vi "RDV-linkPlotSize.vi"(8 "error in (no error)":errorcluster, 11 "RDV-Reflection_Data_viewer in":refnum<class "RDV-Reflection_Data_viewer.lvclass">) -> (0 "error out":errorcluster, 3 "RDV-Reflection_Data_viewer out":refnum<class "RDV-Reflection_Data_viewer.lvclass">)   [LabVIEW 2020, in "RDV-Reflection_Data_viewer.lvclass"]
uses:
  RDV-Reflection_Data_viewer.lvclass
  RDV-Reflection_Data_viewer.lvclass/RDV-Reflection_Data_viewer.ctl
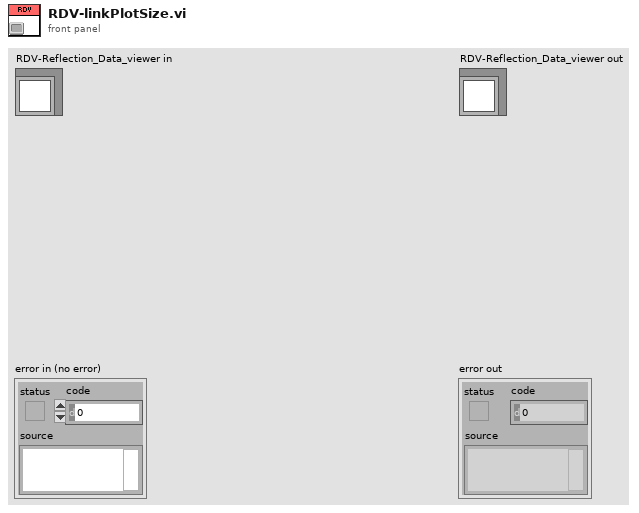
[diagram p1: front panel]
types:
  T1 = typedef "RDV-Reflection_Data_viewer.lvclass/RDV-XY_GRAPH_REFS.ctl" = cluster{"Reflection Real":refnum<vi>, "Reflection Imag":refnum<vi>, "Permittivity Real":refnum<vi>, "Permittivity Imag":refnum<vi>}
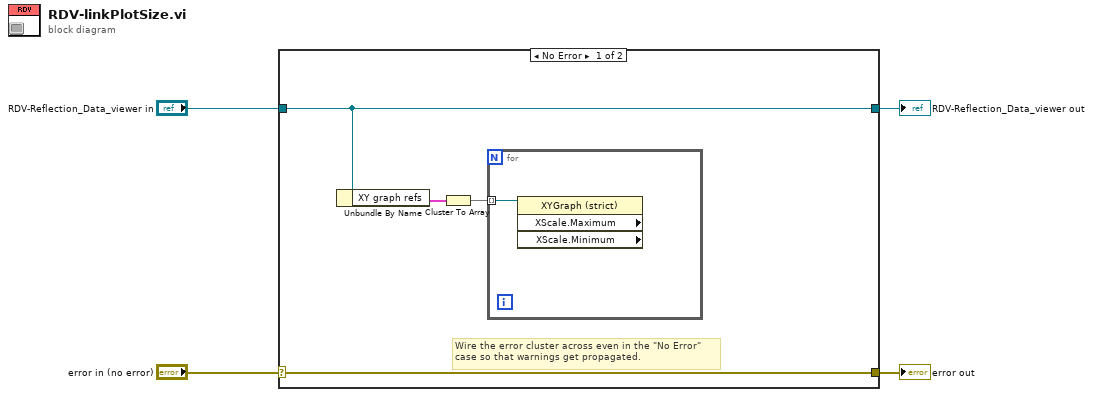
[diagram p0: block diagram]
diagram:
  n1 = case shown="No Error" "error in (no error)" {
    selector: "error in (no error)" -> [w8 w11]
    tunnel: [w8 w11] -> w3
    tunnel: [w7 w10] -> w1
    tunnel: "RDV-Reflection_Data_viewer in" -> [w7 w10]
    frame No Error {
      # "Wire the error cluster across even in the \"No Error\"\ncase so that warnings get propagated."
      n2 = Unbundle By Name(w7) -> ("XY graph refs"=w6:T1)
      n3 = Cluster To Array(cluster=w6) -> (array=w5:refnum<vi>[])
      n4 = for {
        tunnel: w5 -> [w9] mode=indexing
        n5 = property on="Property Node" class="XYGraph (strict)" props=["XScale", "Maximum", "XScale", "Minimum"](reference=w9) -> ()  [unwired: 1 in, 4 out]
      }
    }
    frame Error {
    }
  }
  "error out" <- w3
  "RDV-Reflection_Data_viewer out" <- w1
